vi "tcp_client_meas_time.vi"() -> ()   [LabVIEW 2019]
panel:
  out "TCP Read (ms)":u32(graph)
  out "TCP Open (ms)":u32(graph)
  out "error out":errorcluster
  out "TCP Close (ms)":u32(graph)
  out "status":bool
  out "EOS":bool=TRUE
  out "BOS":bool=TRUE
  out "client_step":i32
  in  "stop_query":bool
  out "spill_id":i32
  # "ASAP Mode"
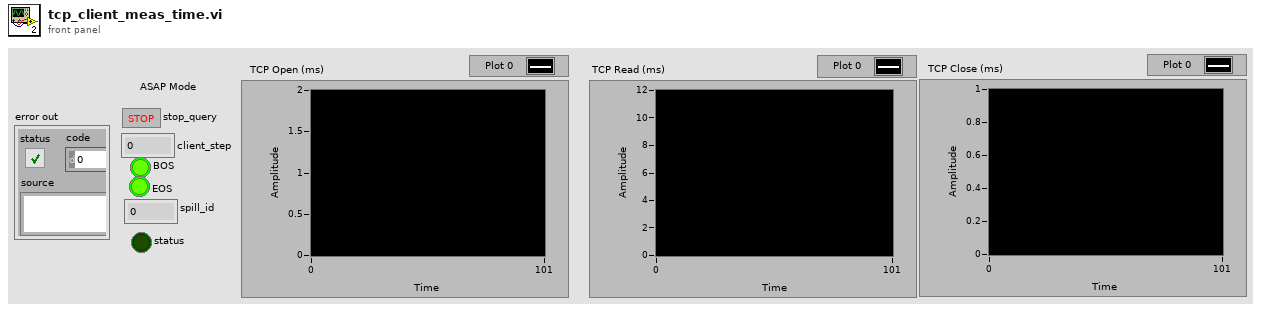
[diagram p1: front panel]
types:
  T1 = enum16{"Standard", "Buffered", "CRLF", "Immediate"}
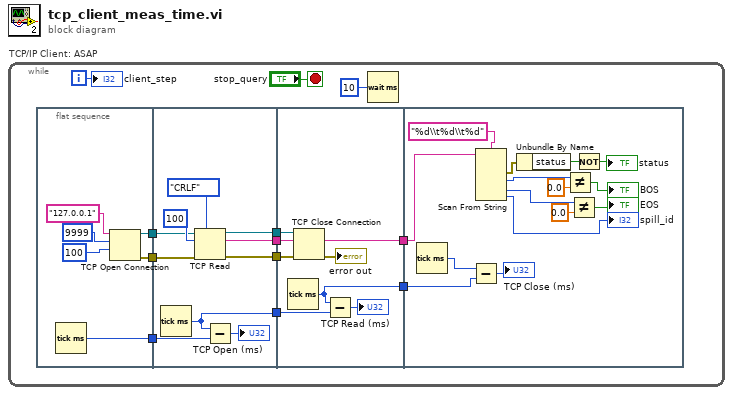
[diagram p0: block diagram]
diagram:
  n1 = while "TCP/IP Client: ASAP" {
    i -> [w10]
    stop <- "stop_query" stop-if-true
    n2 = flat-sequence {
      tunnel: [w18] -> w9
      tunnel: [w14] -> w8
      tunnel: [w13] -> w7
      tunnel: w9 -> [w23]
      tunnel: [w22] -> w6
      tunnel: w8 -> [w26]
      tunnel: w7 -> [w25]
      tunnel: [w21] -> w4
      tunnel: [w20] -> w3
      tunnel: [w19] -> w2
      tunnel: w6 -> [w32]
      tunnel: [w31] -> w5
      tunnel: w4 -> [w29]
      tunnel: w3 -> [w34]
      tunnel: w2 -> [w33]
      tunnel: [w29] -> w1
      tunnel: w5 -> [w49]
      tunnel: w1 -> [w40]
      frame #0 {
        n3 = Tick Count (ms)() -> (millisecond timer value=w18:u32)
        n4 = TCP Open Connection(address="127.0.0.1", remote port or service name=u16 9999 ("port"), timeout ms (60000)=100 ("wait_time")) -> (connection ID=w14:refnum<k5>, error out=w13:errorcluster)  [unwired: 2 in]
      }
      frame #1 {
        n5 = Tick Count (ms)() -> (millisecond timer value=w22:u32)
        n6 = TCP Read(connection ID=w26, bytes to read=100, error in (no error)=w25, 7:T1."CRLF" ("mode (standard)")) -> (connection ID out=w19:refnum<k5>, data out=w21:string, error out=w20:errorcluster)  [unwired: 1 in]
        n7 = Subtract(x=w22, y=w23) -> (x-y=→"TCP Open (ms)":u32)
      }
      frame #2 {
        n8 = Tick Count (ms)() -> (millisecond timer value=w31:u32)
        n9 = TCP Close Connection(connection ID=w33, error in (no error)=w34) -> (error out=→"error out":errorcluster)  [unwired: 1 in, 1 out]
        n10 = Subtract(x=w31, y=w32) -> (x-y=→"TCP Read (ms)":u32)
      }
      frame #3 {
        n11 = Tick Count (ms)() -> (millisecond timer value=w50:u32)
        n12 = Subtract(x=w50, y=w49) -> (x-y=→"TCP Close (ms)":u32)
        n13 = Scan From String(format string="%d\\t%d\\t%d", input string=w40) -> (error out=w47:errorcluster, output 1=w45:i32, output 2=w44:i32, output 3=→"spill_id":i32)  [unwired: 5 in, 2 out]
        n14 = Unbundle By Name(w47) -> ("status"=w46:bool)
        n15 = Not Equal?(x=w45, y=0.0) -> (x != y?=→"BOS":bool)
        n16 = Not Equal?(x=w44, y=0.0) -> (x != y?=→"EOS":bool)
        n17 = Not(x=w46) -> (.not. x?=→"status":bool)
      }
    }
    n18 = Wait (ms)(milliseconds to wait=u32 10) -> ()  [unwired: 1 out]
    "client_step" <- w10
  }
